vi "test Set and Get Properties.vi"(8 "error in (no error)":errorcluster, 11 "TestCase in":refnum<class "SLSC Switch Scripting Unit Tests.lvclass">) -> (0 "error out":errorcluster, 3 "TestCase out":refnum<class "SLSC Switch Scripting Unit Tests.lvclass">)   [LabVIEW 2017, in "SLSC Switch Scripting Unit Tests.lvclass"]
uses:
  SLSC Switch Scripting Unit Tests.lvclass
  <vilib>/addons/_JKI Toolkits/VI Tester/TestCase.llb/TestCase.lvclass
  NI-SWITCH Scripting.lvlib
  Properties/SLSC Switch All Properties.ctl
  Custom Device/Find All SLSC Switch Custom Devices.vi
  Shared/Routing and Faulting Hardware API/Routing and Faulting Hardware API.lvlib
  C:/Program Files (x86)/National Instruments/LabVIEW 2017/vi.lib/addons/_JKI Toolkits/VI Tester/TestCase.llb/TestCase.lvclass
panel:
  in  "Save?":bool
  out "Output Filename":string
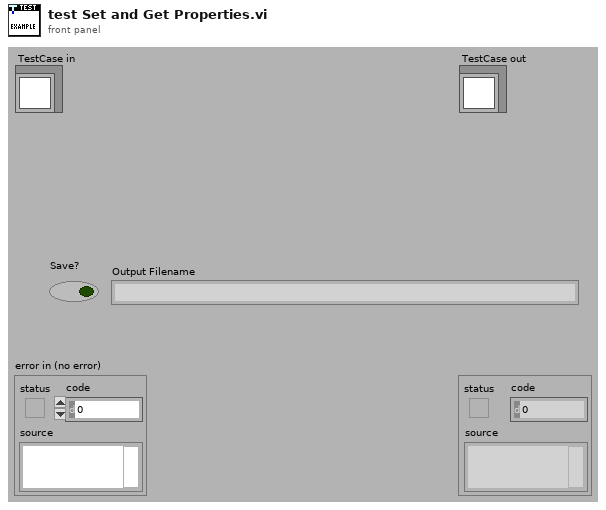
[diagram p1: front panel]
types:
  T1 = typedef "NI-SWITCH Scripting.lvlib/SLSC Switch All Properties.ctl" = cluster{"Product Name":string, "Topology":string, "Switches JSON":string, "Description":string, "Reservation Group":string}
  T2 = typedef "Custom Device API.lvlib/Custom Device Item Ref.ctl" = u64
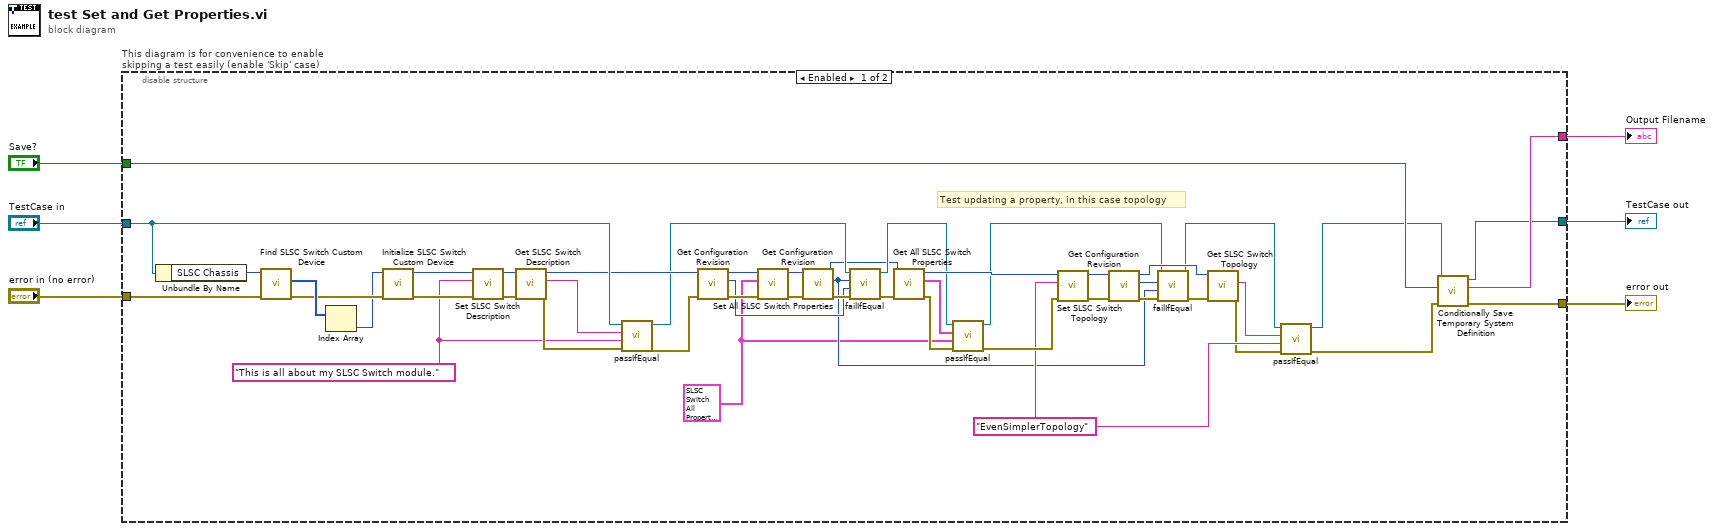
[diagram p0: block diagram]
diagram:
  n1 = disable-structure "This diagram is for convenience to enable skipping a test easily (enable 'Skip' case)" shown="Enabled" {
    disable-tunnel: "TestCase in" -> [w41 w58]
    disable-tunnel: [w52 w56] -> w3
    disable-tunnel: [w53 w57] -> w5
    disable-tunnel: "error in (no error)" -> [w46 w55]
    disable-tunnel: [w54 _] -> w2
    disable-tunnel: "Save?" -> [w51 _]
    frame Enabled {
      w7 = T1 {"Product Name"="Fake Device", "Topology"="SimpleTopology", "Switches JSON"="{\n   \"switchesSpecVersion\": 1,\n   \"relays\": [\n      {\n         \"name\": \"DUT0_LOAD0\",\n         \"actions\": [\n            {\n               \"type\": \"property\",\n               \"resource\": \"Foo\",\n               \"value\": \"Vendor.DUT0_LOAD0\"\n            },\n            {\n               \"type\": \"command\",\n               \"resource\": \"Foo\",\n               \"value\": \"Vendor.Update\"\n            }\n         ]\n      },\n      {\n         \"name\": \"DUT1_LOAD1\",\n         \"actions\": [\n            {\n               \"type\": \"property\",\n               \"resource\": \"Foo\",\n               \"value\": \"Vendor.DUT1_LOAD1\"\n            },\n            {\n               \"type\": \"command\",\n               \"resource\": \"Foo\",\n               \"value\": \"Vendor.Update\"\n            }\n         ]\n      },\n      {\n         \"name\": \"DUT0_DUT1\",\n         \"actions\": [\n            {\n               \"type\": \"property\",\n               \"resource\": \"Foo\",\n               \"value\": \"Vendor.DUT0_DUT1\"\n            },\n            {\n               \"type\": \"command\",\n               \"resource\": \"Foo\",\n               \"value\": \"Vendor.Update\"\n            }\n         ]\n      }\n   ],\n   \"topologies\": [\n      {\n         \"name\": \"SimpleTopology\",\n         \"initialState\": {\n            \"open\": [\n               \"DUT0_LOAD0\",\n               \"DUT1_LOAD1\",\n               \"DUT0_DUT1\"\n            ],\n            \"close\": []\n         },\n         \"channelList\": {\n            \"names\": [\n               \"DUT0\",\n               \"DUT1\",\n               \"LOAD0\",\n               \"LOAD1\"\n            ]\n         },\n         \"connectionList\": [\n            {\n               \"src\": \"DUT0\",\n               \"dest\": \"LOAD0\",\n               \"relays\": [\n                  \"DUT0_LOAD0\"\n               ]\n            },\n            {\n               \"src\": \"DUT1\",\n               \"dest\": \"LOAD1\",\n               \"relays\": [\n                  \"DUT1_LOAD1\"\n               ]\n            },\n            {\n               \"src\": \"DUT0\",\n               \"dest\": \"DUT1\",\n               \"relays\": [\n                  \"DUT0_DUT1\"\n               ]\n            }\n         ]\n      },\n      {\n         \"name\": \"EvenSimplerTopology\",\n         \"initialState\": {\n            \"open\": [\n               \"DUT0_LOAD0\",\n               \"DUT1_LOAD1\"\n            ],\n            \"close\": []\n         },\n         \"channelList\": {\n            \"names\": [\n               \"DUT0\",\n               \"DUT1\",\n               \"LOAD0\",\n               \"LOAD1\"\n            ]\n         },\n         \"connectionList\": [\n            {\n               \"src\": \"DUT0\",\n               \"dest\": \"LOAD0\",\n               \"relays\": [\n                  \"DUT0_LOAD0\"\n               ]\n            },\n            {\n               \"src\": \"DUT1\",\n               \"dest\": \"LOAD1\",\n               \"relays\": [\n                  \"DUT1_LOAD1\"\n               ]\n            }\n         ]\n      }\n   ],\n   \"multiStateRelays\": []\n}", "Description"="my description of this CD", "Reservation Group"="Custom Reservation Group"} ("SLSC Switch All Properties")
      w32 = "EvenSimplerTopology" ("Topology")
      w38 = "This is all about my SLSC Switch module." ("Description")
      # "Test updating a property, in this case topology"
      n2 = Unbundle By Name(w41) -> ("SLSC Chassis"=w47:u64)
      n3 = call-poly "Find SLSC Switch Custom Device.vi"("error in"=w46, "slsc chassis in"=w47) -> ("error out"=w49:errorcluster, "slsc switch custom devices"=w50:T2[])  [unwired: 7 in, 1 out]
      n4 = Index Array(array=w50) -> (element=w48:T2)  [unwired: 1 in]
      n5 = call "Initialize SLSC Switch Custom Device.vi"("error in"=w49, "slsc switch custom device in"=w48) -> ("error out"=w44:errorcluster, "slsc switch custom device out"=w45:T2)  [unwired: 7 in, 1 out]
      n6 = call "Set SLSC Switch Description.vi"("error in"=w44, "description"=w38, "slsc switch custom device in"=w45) -> ("error out"=w39:errorcluster, "slsc switch custom device out"=w43:T2)  [unwired: 7 in]
      n7 = call "Get SLSC Switch Description.vi"("error in"=w39, "slsc switch custom device in"=w43) -> ("error out"=w40:errorcluster, "description"=w42:string, "slsc switch custom device out"=w27:T2)  [unwired: 7 in]
      n8 = call-dynamic "passIfEqual.vi"("error in (no error)"=w40, "y"=w38, "x"=w42, "TestCase in"=w41) -> ("error out"=w25:errorcluster, "TestCase out"=w20:refnum<class "SLSC Switch Scripting Unit Tests.lvclass">)  [unwired: 6 in]
      n9 = call "Get Configuration Revision.vi"("error in (no error)"=w25, "Hardware Ref in"=w27) -> ("error out"=w28:errorcluster, "Configuration Revision"=w17:u32, "Hardware Ref out"=w26:T2)  [unwired: 6 in, 1 out]
      n10 = call "Set All SLSC Switch Properties.vi"("error in"=w28, "properties"=w7, "slsc switch custom device in"=w26) -> ("error out"=w24:errorcluster, "slsc switch custom device out"=w23:T2)  [unwired: 7 in]
      n11 = call "Get Configuration Revision.vi"("error in (no error)"=w24, "Hardware Ref in"=w23) -> ("error out"=w22:errorcluster, "Configuration Revision"=w9:u32, "Hardware Ref out"=w18:T2)  [unwired: 6 in, 1 out]
      n12 = call-dynamic "failIfEqual.vi"("error in (no error)"=w22, "y"=w17, "x"=w9, "TestCase in"=w20) -> ("error out"=w21:errorcluster, "TestCase out"=w19:refnum<class "SLSC Switch Scripting Unit Tests.lvclass">)  [unwired: 6 in]
      n13 = call "Get All SLSC Switch Properties.vi"("error in"=w21, "slsc switch custom device in"=w18) -> ("error out"=w37:errorcluster, "properties"=w36:T1, "slsc switch custom device out"=w35:T2)  [unwired: 7 in]
      n14 = call-dynamic "passIfEqual.vi"("error in (no error)"=w37, "y"=w7, "x"=w36, "TestCase in"=w19) -> ("error out"=w34:errorcluster, "TestCase out"=w12:refnum<class "SLSC Switch Scripting Unit Tests.lvclass">)  [unwired: 6 in]
      n15 = call "Set SLSC Switch Topology.vi"("error in"=w34, "topology"=w32, "slsc switch custom device in"=w35) -> ("error out"=w16:errorcluster, "slsc switch custom device out"=w15:T2)  [unwired: 7 in]
      n16 = call "Get Configuration Revision.vi"("error in (no error)"=w16, "Hardware Ref in"=w15) -> ("error out"=w14:errorcluster, "Configuration Revision"=w10:u32, "Hardware Ref out"=w13:T2)  [unwired: 6 in, 1 out]
      n17 = call-dynamic "failIfEqual.vi"("error in (no error)"=w14, "y"=w9, "x"=w10, "TestCase in"=w12) -> ("error out"=w8:errorcluster, "TestCase out"=w11:refnum<class "SLSC Switch Scripting Unit Tests.lvclass">)  [unwired: 6 in]
      n18 = call "Get SLSC Switch Topology.vi"("error in"=w8, "slsc switch custom device in"=w13) -> ("error out"=w31:errorcluster, "topology"=w33:string)  [unwired: 7 in, 1 out]
      n19 = call-dynamic "passIfEqual.vi"("error in (no error)"=w31, "y"=w32, "x"=w33, "TestCase in"=w11) -> ("error out"=w29:errorcluster, "TestCase out"=w30:refnum<class "SLSC Switch Scripting Unit Tests.lvclass">)  [unwired: 6 in]
      n20 = call "Conditionally Save Temporary System Definition.vi"("error in (no error)"=w29, "Save?"=w51, "Test Case"=w30) -> ("error out"=w53:errorcluster, "filename"=w54:string, "Test Case"=w52:refnum<class "SLSC Switch Scripting Unit Tests.lvclass">)  [unwired: 6 in]
    }
    frame Disabled {
      # "skip test result while test is under development"
      n21 = call <vilib>:"skip.vi"("error in (no error)"=w55, "TestCase in"=w58) -> ("error out"=w57:errorcluster, "TestCase out"=w56:refnum<class "SLSC Switch Scripting Unit Tests.lvclass">)  [unwired: 8 in]
    }
  }
  "error out" <- w5
  "TestCase out" <- w3
  "Output Filename" <- w2
